vi "seleciona_tempo_inicio.vi"(2 "teste":string, 3 "file path (dialog if empty)":path) -> (0 "time_UDP":dbl format="%#_12f", 1 "time_NI":dbl format="%#_12f")   [LabVIEW 2019]
doc: "Input: Faz a leitura do arquivo de entrada, procura por um determinado conjunto de dados indexados pelo nome do teste. \n\nOutput: Retorna as velocidades de início de aquisição NI e UDP"
uses:
  <vilib>/Utility/file.llb/Read Delimited Spreadsheet (string).vi
panel:
  out "pos":i32
  out "arquivo inteiro":string[][](array[string])
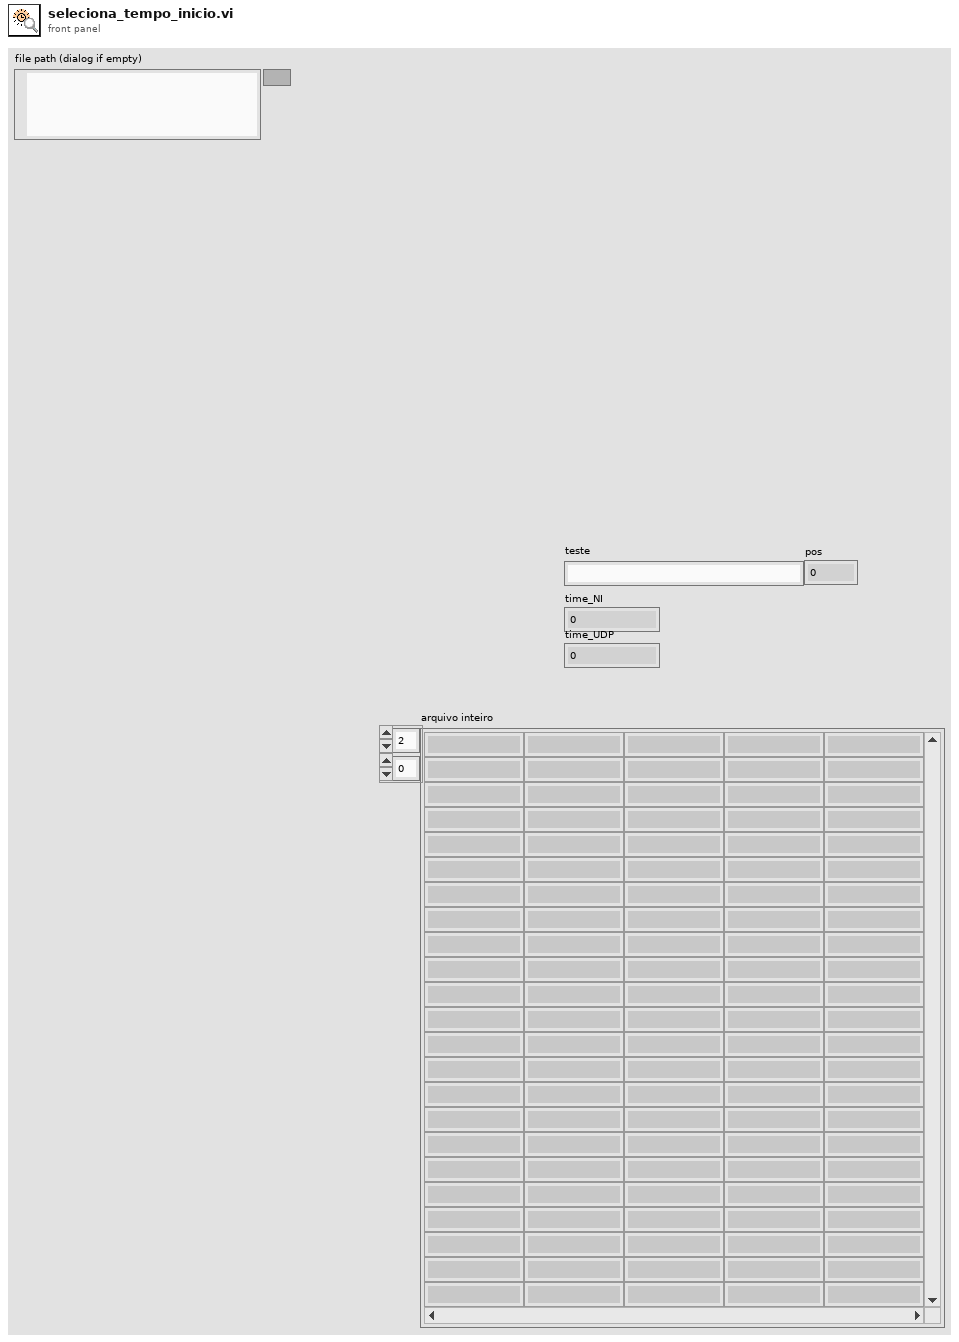
[diagram p1: front panel]
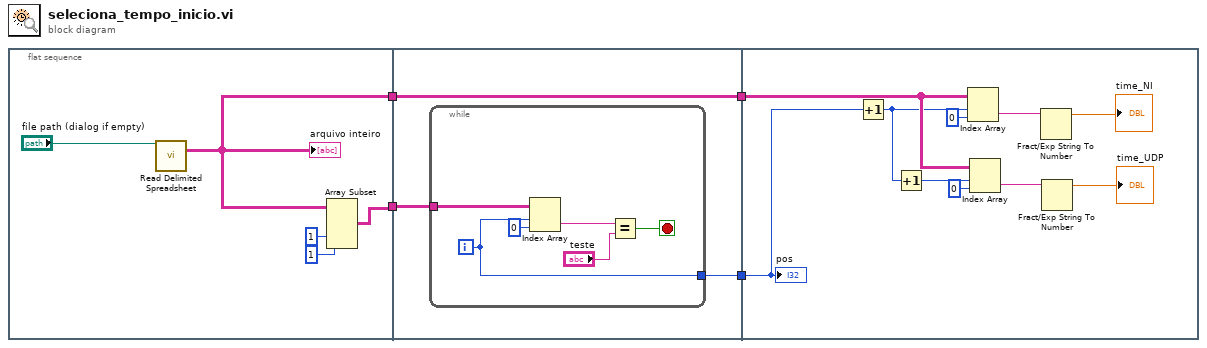
[diagram p0: block diagram]
diagram:
  n1 = flat-sequence {
    tunnel: [w7] -> w4
    tunnel: [w6] -> w2
    tunnel: w4 -> [w12]
    tunnel: [w11] -> w3
    tunnel: w2 -> [w10]
    tunnel: [w10] -> w1
    tunnel: w3 -> [w28]
    tunnel: w1 -> [w25]
    frame #0 {
      n2 = call-poly <vilib>:"Read Delimited Spreadsheet.vi"("file path (dialog if empty)"="file path (dialog if empty)") -> ("all rows"=w6:string[][])  [unwired: 9 in, 5 out]
      "arquivo inteiro" <- w6
      n3 = Array Subset(array=w6, index (col)=1 ("index"), length (col)=1 ("length")) -> (w7:string[][])  [unwired: 2 in]
    }
    frame #1 {
      n4 = while {
        tunnel: w12 -> [w18]
        tunnel: [w13] -> w11
        i -> [w13]
        stop <- w14 stop-if-true
        n5 = Index Array(array=w18, index (row)=w13, index (col)=0 ("disabled index (col)")) -> (element=w16:string)
        n6 = Equal?(x=w16, y="teste") -> (x = y?=w14:bool)
      }
    }
    frame #2 {
      n7 = Increment(x=w28) -> (x+1=w23:i32)
      n8 = Increment(x=w23) -> (x+1=w24:i32)
      n9 = Index Array(array=w25, index (row)=w23, index (col)=0 ("disabled index (col)")) -> (element=w22:string)
      n10 = Index Array(array=w25, index (row)=w24, index (col)=0 ("disabled index (col)")) -> (element=w21:string)
      n11 = Fract/Exp String To Number(string=w22) -> (number=→"time_NI":dbl)  [unwired: 3 in, 1 out]
      n12 = Fract/Exp String To Number(string=w21) -> (number=→"time_UDP":dbl)  [unwired: 3 in, 1 out]
      "pos" <- w28
    }
  }
